vi "matlab_test1.vi"() -> ()   [LabVIEW 2025]
panel:
  in  "reset":bool
  in  "x":dbl
  in  "stop":bool
  out "x out":dbl
  out "error out":errorcluster
  out "Real":dbl
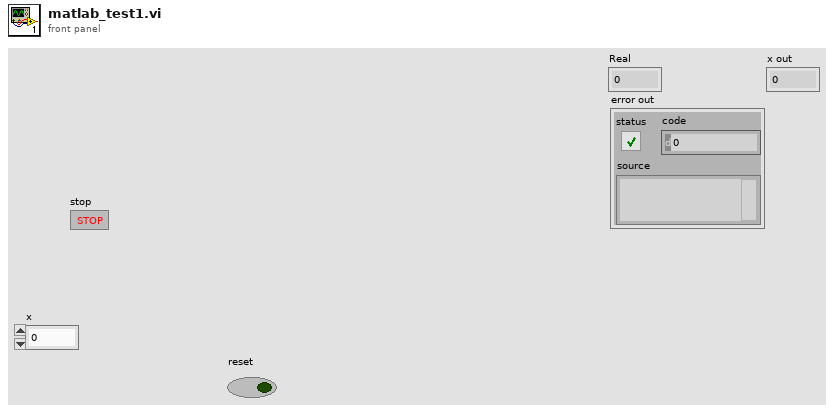
[diagram p1: front panel]
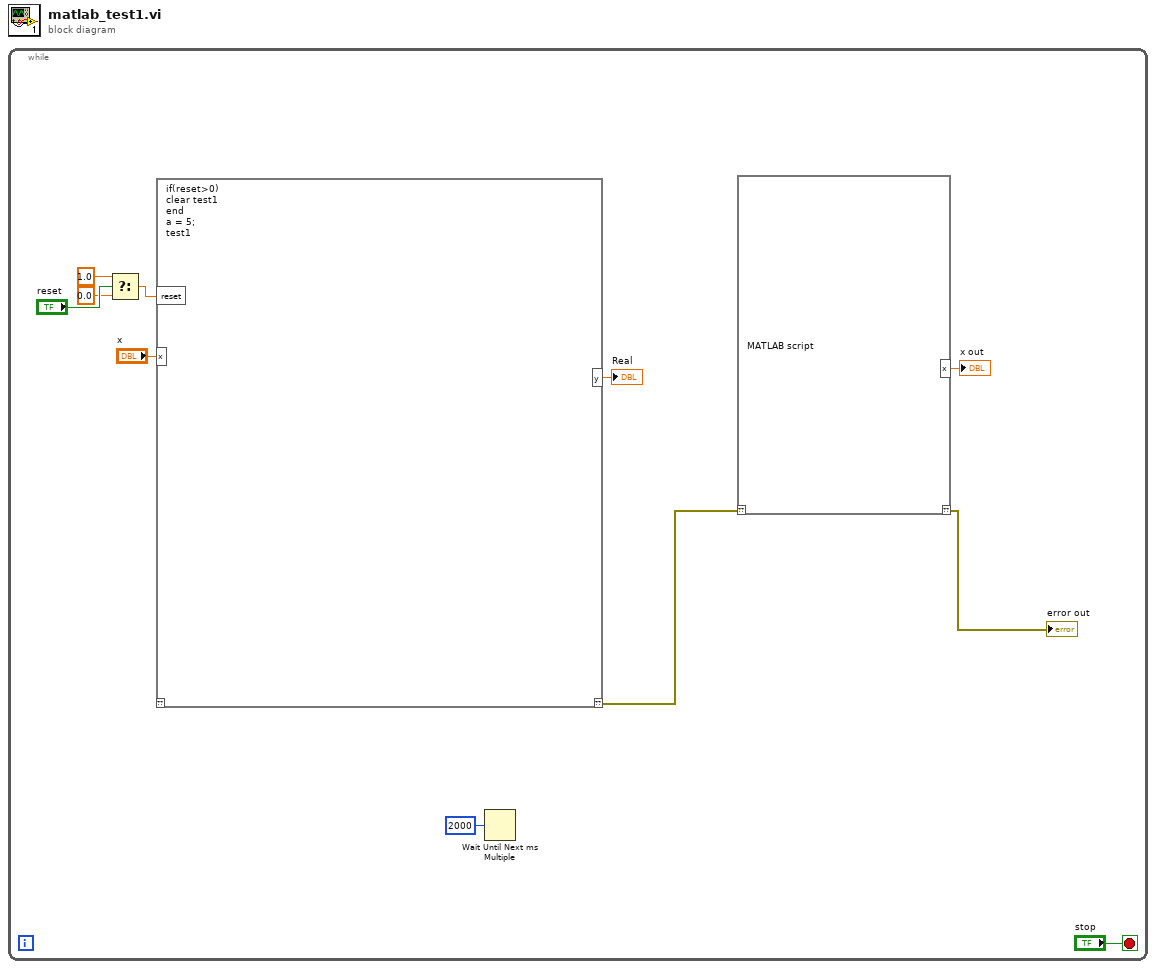
[diagram p0: block diagram]
diagram:
  n1 = while {
    stop <- "stop" stop-if-true
    n2 = Select(t=1.0, s="reset", f=0.0) -> (s? t:f=w1:dbl)
    n3 = script code="if(reset>0)\nclear test1\nend\na = 5;\ntest1"("x"="x", "reset"=w1) -> ("??"=w10:errorcluster, "y"=→"Real":dbl)  [unwired: 1 in]
    n4 = Wait Until Next ms Multiple(millisecond multiple=u32 2000) -> ()  [unwired: 1 out]
    n5 = script code="MATLAB script"("??"=w10) -> ("??"=→"error out":errorcluster, "x"=→"x out":dbl)
  }
